vi "LED Strip Lights.vi"() -> ()   [LabVIEW 2025]
doc: "This example shows how to write to addressable LED strip lights.\n\nThis example expects a USB cable connected from your development PC to the Type B USB Jack (next to the power input) on the roboRIO."
uses:
  <vilib>/Rock Robotics/SystemInterfaces/DIO/FPGA_DIOPWMChannel.ctl
panel:
  in  "PWM Channel":T1=enum."PWM 9"
  out "LED Strip":u32[](array[colorbox])
  in  "String Length":u16=8
  in  "stop":bool
  # "Set this input before running."
  # "This shows the colors sent."
  # "LED Strip Lights"
  # "This shows wiring for an addressable LED Strip Light. Only one light strip is supported on the roboRIO. Controls WS2812B and compatible strips."
  # "DIN"
  # "+5V"
  # "GND"
  # "^"
  # "^"
  # "^"
  # "^"
  # "LED Strip\nDIN (blue wire)-------\n+5V (red wire)--------\nGND (black wire)-----"
  # "roboRIO\nPWM-9  S \nPWM-9  V\nPWM-9"
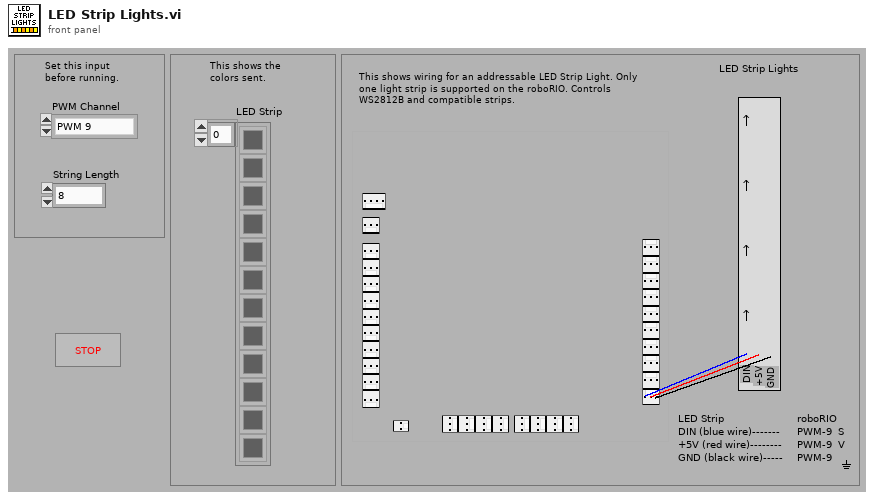
[diagram p1: front panel]
types:
  T1 = typedef "FPGA_DIOPWMChannel.ctl" = enum8{"PWM 0", "PWM 1", "PWM 2", "PWM 3", "PWM 4", "PWM 5", "PWM 6", "PWM 7", "PWM 8", "PWM 9", "PWM MXP 0", "PWM MXP 1", "PWM MXP 2", "PWM MXP 3", "PWM MXP 4", "PWM MXP 5", "PWM MXP 6", "PWM MXP 7", "PWM MXP 8", "PWM MXP 9", "Invalid"}
  T2 = typedef "WPI_PWMDeviceRef.ctl" = cluster{"DeviceStatus":errorcluster, "PWM Channel":T1}
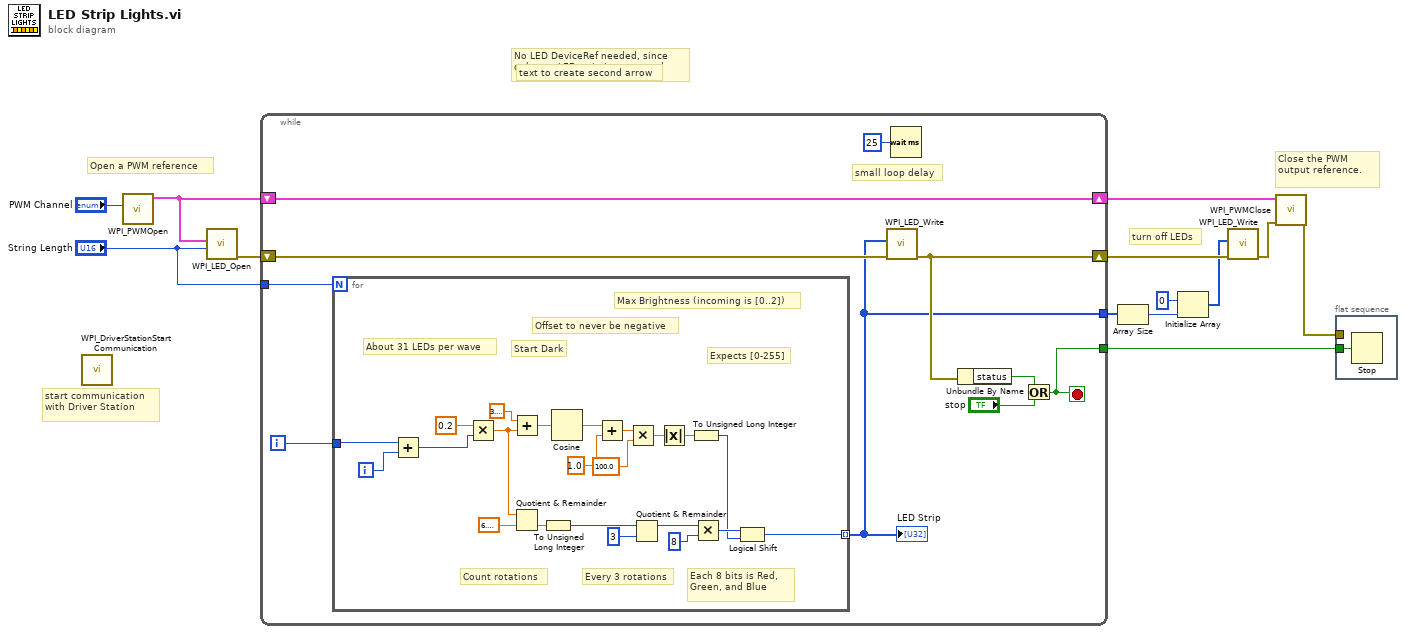
[diagram p0: block diagram]
diagram:
  # "turn off LEDs"
  # "No LED DeviceRef needed, since only one LED strip is supported"
  # "Open a PWM reference"
  # "start communication with Driver Station"
  # "Close the PWM output reference."
  # "text to create second arrow"
  n1 = call <vilib>:"WPI_DriverStationStart Communication.vi"() -> ()  [unwired: 3 in, 9 out]
  n2 = call <vilib>:"WPI_PWMOpen.vi"("PWM Channel"="PWM Channel") -> ("PWMDeviceRef"=w10:T2)  [unwired: 9 in, 1 out]
  n3 = call <vilib>:"WPI_LED_Open.vi"("String Length"="String Length", "PWMDeviceRef"=w10) -> ("error out"=w11:errorcluster)  [unwired: 9 in]
  n4 = while {
    shift-right: [w19] -> w12
    shift-left: w10 -> [w19]
    tunnel: [w22] -> w13
    shift-right: [w17] -> w7
    shift-left: w11 -> [w18]
    tunnel: "String Length" -> [w15]
    tunnel: [w14] -> w4
    i -> [w16]
    stop <- w22 stop-if-true
    # "small loop delay"
    n5 = for {
      N: w15 -> [_]
      tunnel: w16 -> [w44]
      tunnel: [w24] -> w14 mode=indexing
      i -> [w45]
      # "Expects [0-255]"
      # "Max Brightness (incoming is [0..2])"
      # "Offset to never be negative"
      # "About 31 LEDs per wave"
      # "Start Dark"
      # "Each 8 bits is Red, Green, and Blue"
      # "Every 3 rotations"
      # "Count rotations"
      n6 = Add(x=w44, y=w45) -> (x+y=w25:i32)
      n7 = Multiply(x=0.2, y=w25) -> (x*y=w43:dbl)
      n8 = Add(x=3.141592653589793, y=w43) -> (x+y=w37:dbl)
      n9 = Quotient & Remainder(x=w43, y=6.283185307179586) -> (floor(x/y)=w39:dbl)  [unwired: 1 out]
      n10 = To Unsigned Long Integer(number=w39) -> (unsigned 32bit integer=w40:u32)
      n11 = Cosine(x=w37) -> (cos(x)=w34:dbl)
      n12 = Add(x=w34, y=1.0 ("x")) -> (x+y=w33:dbl)
      n13 = Multiply(x=w33, y=100.0 ("x")) -> (x*y=w36:dbl)
      n14 = Quotient & Remainder(x=w40, y=u32 3) -> (x-y*floor(x/y)=w38:u32)  [unwired: 1 out]
      n15 = Absolute Value(x=w36) -> (abs(x)=w35:dbl)
      n16 = To Unsigned Long Integer(number=w35) -> (unsigned 32bit integer=w41:u32)
      n17 = Multiply(x=w38, y=u32 8) -> (x*y=w42:u32)
      n18 = Logical Shift(y=w42, x=w41) -> (x << y=w24:u32)
    }
    "LED Strip" <- w14
    n19 = call <vilib>:"WPI_LED_Write.vi"("error in"=w18, "Color Array"=w14) -> ("error out"=w17:errorcluster)  [unwired: 9 in]
    n20 = Wait (ms)(milliseconds to wait=u32 25) -> ()  [unwired: 1 out]
    n21 = Unbundle By Name(w17) -> ("status"=w20:bool)
    n22 = Or(x=w20, y="stop") -> (x .or. y?=w22:bool)
  }
  n23 = Array Size(array=w4) -> (size(s)=w5:i32)
  n24 = Initialize Array(u32 0, w5) -> (w2:u32[])
  n25 = call <vilib>:"WPI_LED_Write.vi"("error in"=w7, "Color Array"=w2) -> ("error out"=w6:errorcluster)  [unwired: 9 in]
  n26 = call <vilib>:"WPI_PWMClose.vi"("error in (no error)"=w6, "PWMDeviceRef"=w12) -> ("error out"=w1:errorcluster)  [unwired: 9 in]
  n27 = flat-sequence {
    tunnel: w13 -> [w46]
    tunnel: w1 -> [_]
    frame #0 {
      n28 = Stop(stop? (T)=w46) -> ()
    }
  }
